vi "PLCCtrl.vi"(4 "Turn Fans On":bool, 5 "Clear Faults":bool, 6 "Enable Fans":bool, 7 "FanSetpoint_uint":dbl[](array[numeric]), 8 "Error In":errorcluster, 9 "Ctrl Signals In":T1, 10 "PLCInputSignals In":T2, 11 "IO Signals In":T3) -> (0 "Error Out":errorcluster, 1 "Ctrl Signals Out":T1, 2 "PLCInputSignals Out":T2, 3 "IO Signals Out":T3)   [LabVIEW 2018]
uses:
  Clusters/IOSignals.ctl
  Clusters/PLCSignals.ctl
  Clusters/CtrlSignals.ctl
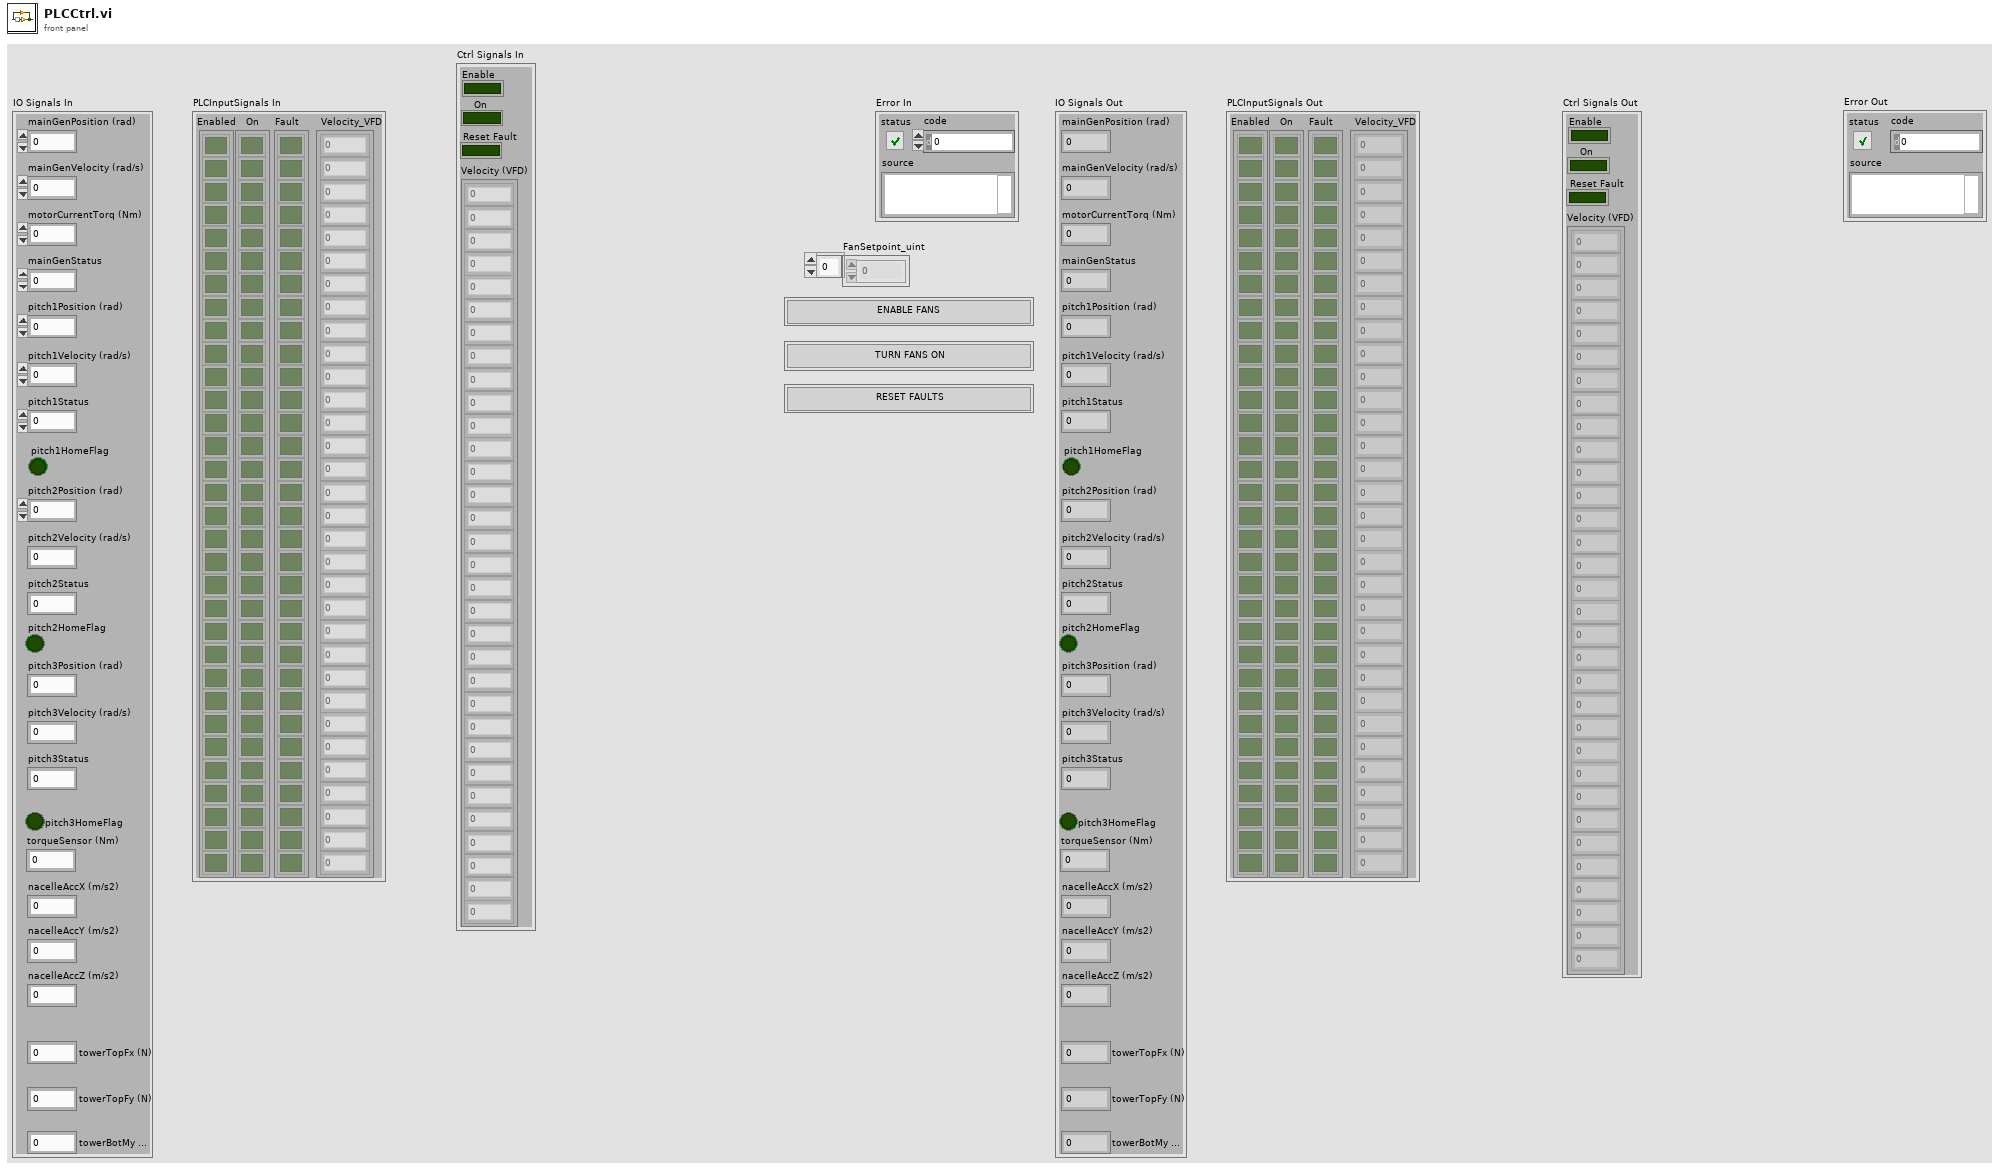
[diagram p1: front panel]
types:
  T1 = typedef "CtrlSignals.ctl" = cluster{"Enable":bool, "On":bool, "Reset Fault":bool, "Velocity (VFD)":i32[]}
  T2 = typedef "PLCSignals.ctl" = cluster{"Enabled":bool[], "On":bool[], "Fault":bool[], "Velocity_VFD":i32[]}
  T3 = typedef "IOSignals.ctl" = cluster{"mainGenPosition (rad)":dbl, "motorCurrentTorq (Nm)":dbl, "mainGenVelocity (rad/s)":dbl, "mainGenStatus":u16, "pitch1Position (rad)":dbl, "pitch1Velocity (rad/s)":dbl, "pitch1Status":u16, "pitch2Position (rad)":dbl, "pitch2Velocity (rad/s)":dbl, "pitch2Status":u16, "pitch3Position (rad)":dbl, "pitch3Velocity (rad/s)":dbl, "pitch3Status":u16, "torqueSensor (Nm)":dbl, "nacelleAccX (m/s2)":dbl, "nacelleAccY (m/s2)":dbl, "nacelleAccZ (m/s2)":dbl, "pitch1HomeFlag":bool, "pitch2HomeFlag":bool, "pitch3HomeFlag":bool, "towerTopFx (N)":dbl, "towerTopFy (N)":dbl, "towerBotMy (Nm)":dbl}
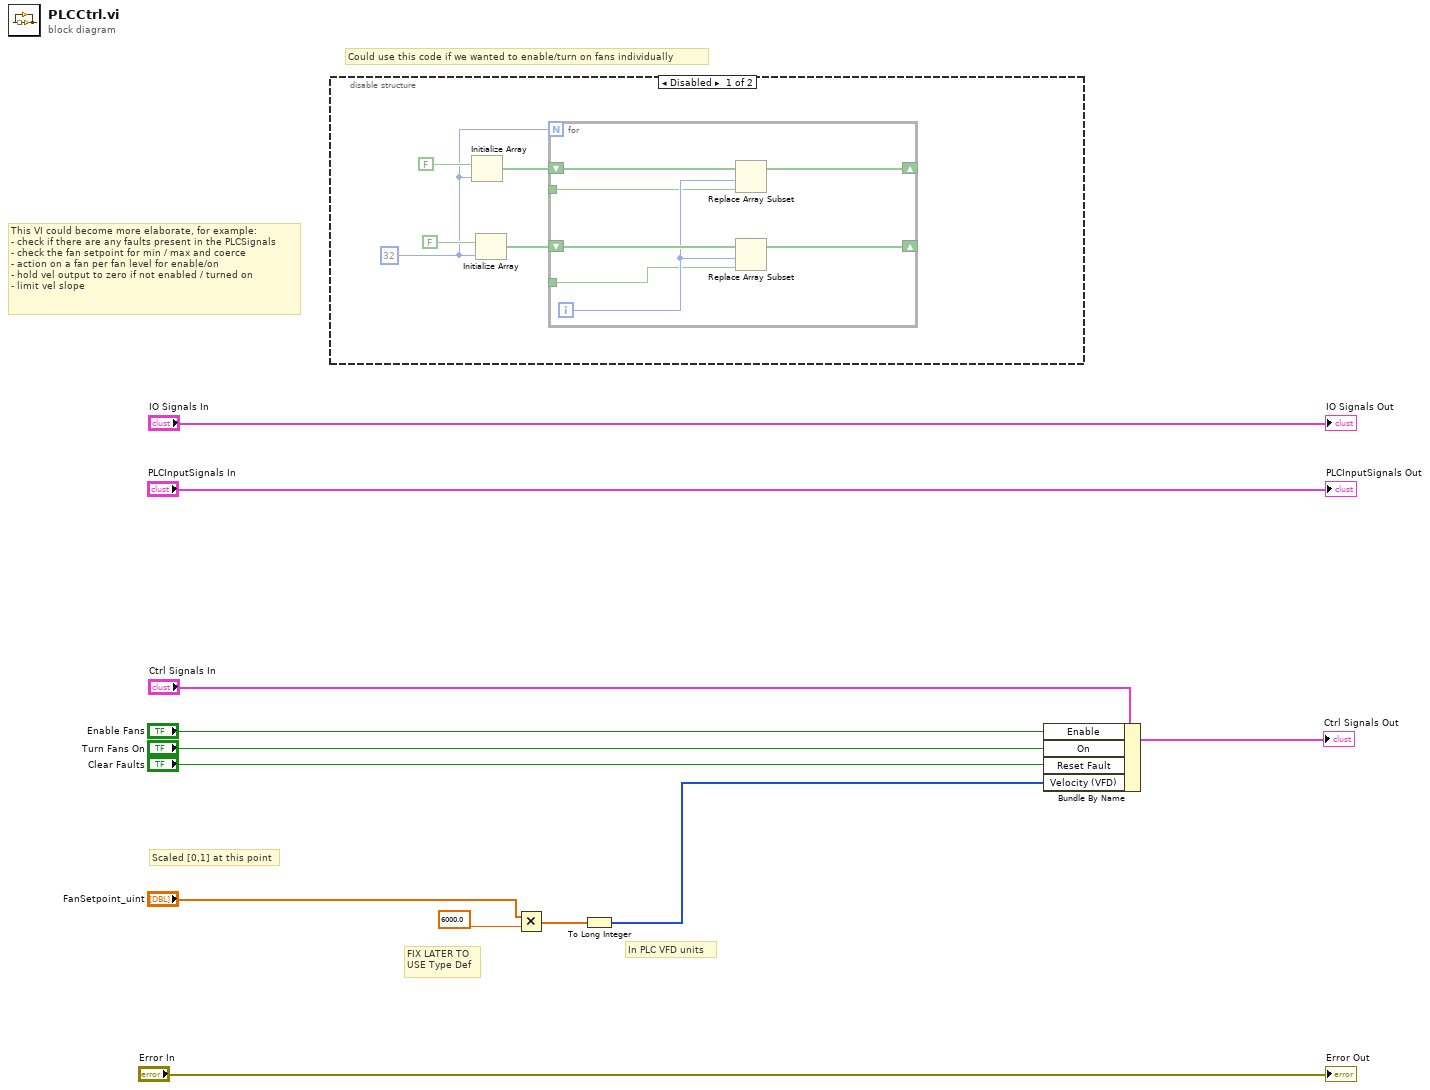
[diagram p0: block diagram]
diagram:
  # "FIX LATER TO\nUSE Type Def"
  # "In PLC VFD units"
  # "Scaled [0,1] at this point"
  # "This VI could become more elaborate, for example:\n- check if there are any faults present in the PLCSignals\n- check the fan setpoint for min / max and coerce\n- action on a fan per fan level for enable/on\n- hold vel output to zero if not enabled / turned on\n- limit vel slope"
  # "Could use this code if we wanted to enable/turn on fans individually"
  n1 = disable-structure shown="Disabled" {
    frame Disabled {
      w15 = 32 ("dimension size")
      n2 = Initialize Array(FALSE, w15) -> (w14:bool[])
      n3 = Initialize Array(FALSE, w15) -> (w13:bool[])
      n4 = for {
        N: w15 -> [_]
        shift-right: [w19] -> _
        shift-left: w14 -> [w24]
        shift-right: [w18] -> _
        shift-left: w13 -> [w23]
        tunnel: _ -> [w21]
        tunnel: _ -> [w20]
        i -> [w22]
        n5 = Replace Array Subset(array=w24, new element=w21, index=w22) -> (w19:bool[])
        n6 = Replace Array Subset(array=w23, new element=w20, index=w22) -> (w18:bool[])
      }
    }
    frame Enabled {
    }
  }
  n7 = Multiply(x="FanSetpoint_uint", y=6000.0) -> (x*y=w6:dbl[])
  n8 = To Long Integer(number=w6) -> (32bit integer=w5:i32[])
  n9 = Bundle By Name(cluster="Ctrl Signals In", "Enable"="Enable Fans", "On"="Turn Fans On", "Reset Fault"="Clear Faults", "Velocity (VFD)"=w5) -> (→"Ctrl Signals Out":T1)
  "IO Signals Out" <- "IO Signals In"
  "PLCInputSignals Out" <- "PLCInputSignals In"
  "Error Out" <- "Error In"
